vi "Do.vi"(6 "Data":T1[](array[typedef])=[{"Active"=FALSE, "MotorN"=enum."M12"}, {"Active"=FALSE, "MotorN"=enum."M21"}, {"Active"=FALSE, "MotorN"=enum."M24"}], 8 "error in (no error)":errorcluster, 10 "Do":bool, 11 "PM_Group in":refnum<class "PM_Group.lvclass">) -> (0 "error out":errorcluster, 2 "Done":bool, 3 "PM_Group out":refnum<class "PM_Group.lvclass">)   [LabVIEW 2019, in "PM_Group.lvclass"]
uses:
  PM_Group.lvclass
  TypeDef/Active Motor.ctl
  TypeDef/Motor N.ctl
  PM_Group.lvclass/PM_Group.ctl
  Device_class/Device.lvclass/Device.ctl
  Engine_1DO_2DI_class/Engine_1DO_2DI.lvclass/Engine_1DO_2DI.ctl
  Engine_1DO_2DI_class/GetEngineState.vi
  Device_class/GetFPGA.vi
  Engine_1DO_2DI_class/Engine_1DO_2DI.lvclass
  D:/GIT H4000/H4000/src/Device_class/Device.lvclass
  FPGA_API_class/FPGA API.lvclass
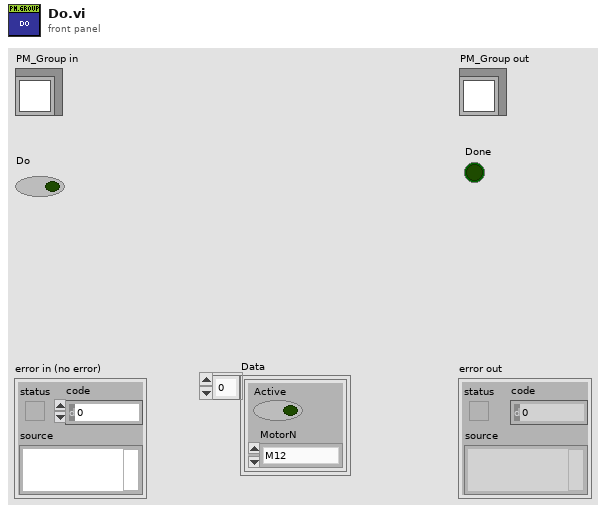
[diagram p1: front panel]
types:
  T1 = typedef "Active Motor.ctl" = cluster{"Active":bool, "MotorN":T2}
  T2 = typedef "Motor N.ctl" = enum16{"M12", "M21", "M24"}
  T3 = typedef "State PMG.ctl" = cluster{"PMG Mode":T4, "M12":T5, "M21":T5, "M24":T5}
  T4 = typedef "PMG Mode.ctl" = enum16{"Idel", "Filling", "Pressure"}
  T5 = typedef "State Engine 2.ctl" = cluster{"EngState":T6, "Active":bool, "Contactor":bool, "CMD":bool, "Automat":bool}
  T6 = typedef "State Engine.ctl" = enum16{"Unknown", "Off", "TupningOn", "On", "TurningOff"}
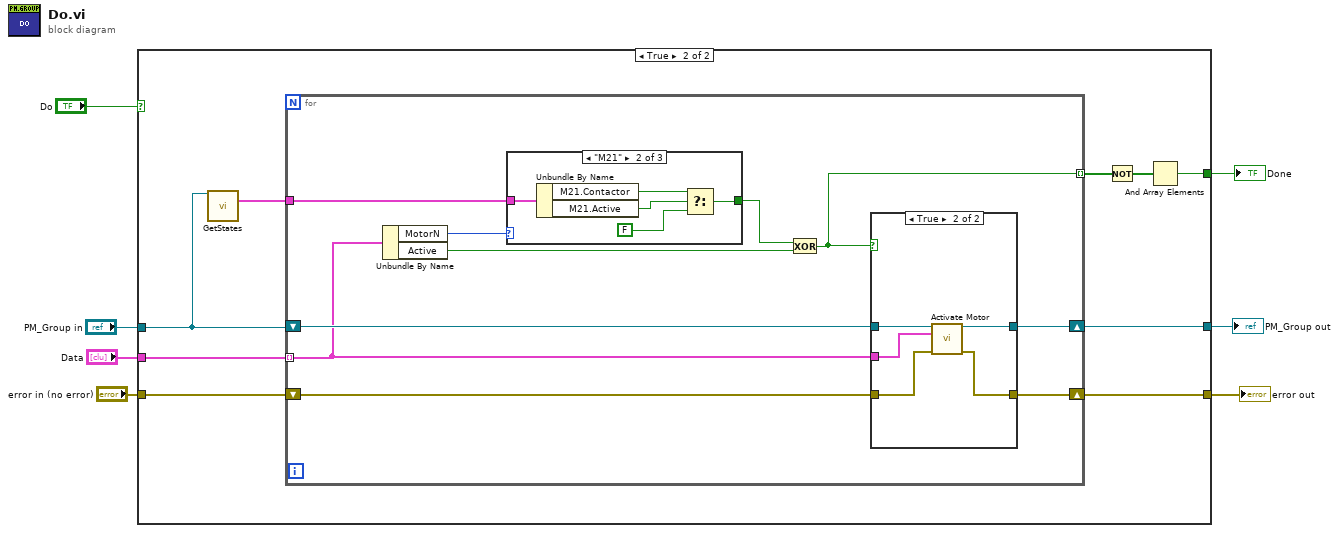
[diagram p0: block diagram]
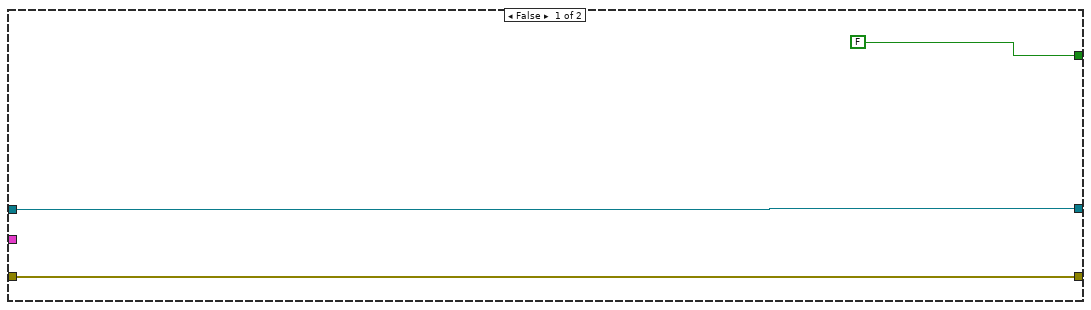
[diagram p2: hidden frame]
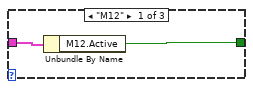
[diagram p4: hidden frame]
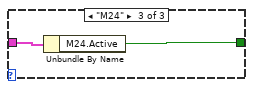
[diagram p5: hidden frame]
diagram:
  n1 = case shown="True" "Do" {
    tunnel: "error in (no error)" -> [w9 w19]
    tunnel: [w9 w18] -> w6
    tunnel: "PM_Group in" -> [w10 w15]
    tunnel: [w10 w17] -> w4
    tunnel: "Data" -> [_ w16]
    tunnel: [FALSE w11] -> w1
    frame False {
    }
    frame True {
      n2 = call "GetStates.vi"("Pump_1AI_1DO_2DI in"=w15) -> ("PMG"=w14:T3)  [unwired: 13 in, 1 out]
      n3 = for {
        tunnel: w16 -> [w25] mode=indexing
        shift-right: [w27] -> w17
        shift-left: w15 -> [w29]
        shift-right: [w26] -> w18
        shift-left: w19 -> [w28]
        tunnel: w14 -> [w24]
        tunnel: [w21] -> w13 mode=indexing
        n4 = Unbundle By Name(w25) -> ("MotorN"=w20:T2, "Active"=w22:bool)
        n5 = case shown="\"M21\"" w20 {
          tunnel: w24 -> [w38 w43 w45]
          tunnel: [w37 w39 w44] -> w23
          frame "M12" {
            n6 = Unbundle By Name(w38) -> ("M12.Active"=w37:bool)
          }
          frame "M21" {
            n7 = Unbundle By Name(w43) -> ("M21.Contactor"=w41:bool, "M21.Active"=w42:bool)
            n8 = Select(t=w41, s=w42, f=FALSE) -> (s? t:f=w39:bool)
          }
          frame "M24" {
            n9 = Unbundle By Name(w45) -> ("M24.Active"=w44:bool)
          }
        }
        n10 = Exclusive Or(1:w22, 2:w23) -> (0:w21:bool)
        n11 = case shown="True" w21 {
          tunnel: w29 -> [w31 w36]
          tunnel: w28 -> [w30 w35]
          tunnel: [w31 w34] -> w27
          tunnel: [w30 w33] -> w26
          tunnel: w25 -> [_ w32]
          frame False {
          }
          frame True {
            n12 = call "Activate Motor.vi"("reference in"=w36, "Active Motor"=w32, "error in (no error)"=w35) -> ("reference out"=w34:refnum<class "PM_Group.lvclass">, "error out"=w33:errorcluster)  [unwired: 11 in]
          }
        }
      }
      n13 = Not(x=w13) -> (.not. x?=w12:bool[])
      n14 = And Array Elements(Boolean array=w12) -> (logical AND=w11:bool)
    }
  }
  "error out" <- w6
  "PM_Group out" <- w4
  "Done" <- w1
